vi "Get User Configuration File.vi"(8 "error in (no error)":errorcluster) -> (0 "error out":errorcluster, 3 "Config":T1)   [LabVIEW 2015]
uses:
  Config/User Configuration.ctl
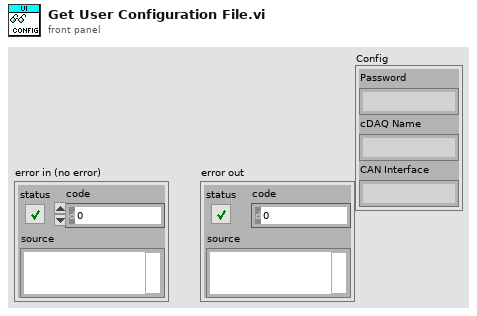
[diagram p1: front panel]
types:
  T1 = typedef "User Configuration.ctl" = cluster{"Password":string, "cDAQ Name":string, "CAN Interface":string}
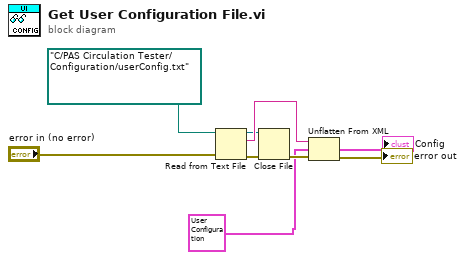
[diagram p0: block diagram]
diagram:
  n1 = Read from Text File(file (use dialog)=path "C:/PAS Circulation Tester/Configuration/userConfig.txt", error in="error in (no error)") -> (refnum out=w6:refnum<file>, text=w7:string, error out=w5:errorcluster)  [unwired: 2 in, 1 out]
  n2 = Close File(refnum=w6, error in=w5) -> (error out=w8:errorcluster)  [unwired: 1 out]
  n3 = Unflatten From XML(xml string=w7, type=T1 {"Password"="admin", "cDAQ Name"="cDAQ9188-1A2B7A8", "CAN Interface"=""} ("User Config"), error in (no error)=w8) -> (value=→"Config":T1, error out=→"error out":errorcluster)
